vi "Close.vi"(0 "PM Simulated in":refnum<class "Simulated Power Meter.lvclass">, 11 "error in (no error)":errorcluster) -> (4 "PM Simulated out":refnum<class "Simulated Power Meter.lvclass">, 15 "error out":errorcluster)   [LabVIEW 2023, in "RFFixtureCharact.Instruments.lvlib" / "Simulated Power Meter.lvclass"]
uses:
  Simulated Power Meter.lvclass
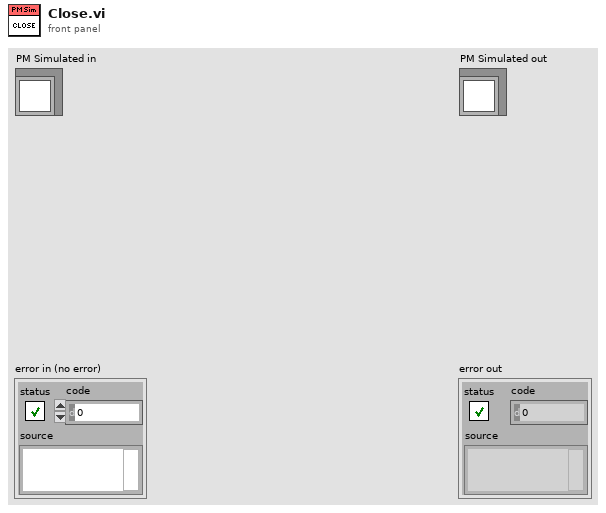
[diagram p1: front panel]
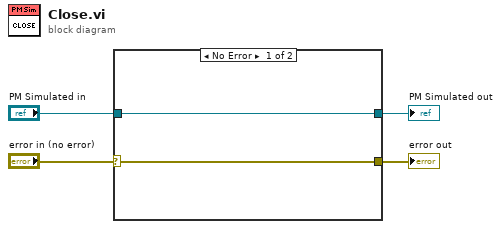
[diagram p0: block diagram]
diagram:
  n1 = case shown="No Error" "error in (no error)" {
    selector: "error in (no error)" -> [w6 w7]
    tunnel: [w6 w7] -> w3
    tunnel: "PM Simulated in" -> [w5 w8]
    tunnel: [w5 w8] -> w1
    frame No Error {
    }
    frame Error {
    }
  }
  "error out" <- w3
  "PM Simulated out" <- w1
